vi "Elevator.vi"(8 "actuating axis":dbl, 11 "Elevator Locked?":bool) -> ()   [LabVIEW 2014]
uses:
  Robot Global Data.vi
panel:
  out "Winch Setpoint":dbl
  out "Winch Motor speed":dbl
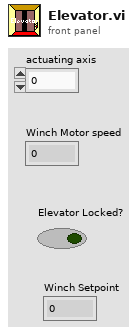
[diagram p1: front panel]
types:
  T1 = typedef "WPI_DigitalInputDevRef.ctl" = cluster{"DevStatus":errorcluster, "DIO Channel":T2, "Controller":T3}
  T2 = typedef "FPGA_DIOChannel.ctl" = enum8{"DIO 0", "DIO 1", "DIO 2", "DIO 3", "DIO 4", "DIO 5", "DIO 6", "DIO 7", "DIO 8", "DIO 9", "DIO MXP 0", "DIO MXP 1", "DIO MXP 2", "DIO MXP 3", "DIO MXP 4", "DIO MXP 5", "DIO MXP 6", "DIO MXP 7", "DIO MXP 8", "DIO MXP 9", "DIO MXP 10", "DIO MXP 11", "DIO MXP 12", "DIO MXP 13", "DIO MXP 14", "DIO MXP 15", "Invalid"}
  T3 = typedef "FPGA_TypedefDigitalModule.ctl" = enum16{"Controller 1"}
  T4 = typedef "WPI_MotorControlDeviceRef.ctl" = cluster{"DeviceStatus":errorcluster, "Type":T5, "PWM":cluster{"Controller":T3, "PWM Channel":T6, "DeadBand":T7}, "CAN":cluster{"Device Number":u8, "Control Mode":T8, "Semaphore":T9, "Max Vout":dbl, "TalonSRX Control Mode":T10}, "Invert":bool, "TransformRef":T11, "InvTransformRef":T11}
  T5 = typedef "WPI_MotorControlType.ctl" = enum16{"PWM", "CAN", "CANTalonSRX"}
  T6 = typedef "FPGA_DIOPWMChannel.ctl" = enum8{"PWM 0", "PWM 1", "PWM 2", "PWM 3", "PWM 4", "PWM 5", "PWM 6", "PWM 7", "PWM 8", "PWM 9", "PWM MXP 0", "PWM MXP 1", "PWM MXP 2", "PWM MXP 3", "PWM MXP 4", "PWM MXP 5", "PWM MXP 6", "PWM MXP 7", "PWM MXP 8", "PWM MXP 9", "Invalid"}
  T7 = typedef "WPI_PWMDeadband.ctl" = cluster{"Name":string, "maxPositivePwm":i32, "minPositivePwm":i32, "centerPwm":i32, "maxNegativePwm":i32, "minNegativePwm":i32, "angularRange":u16}
  T8 = typedef "WPI_CANJaguar_ControlMode.ctl" = enum8{"Percent VBus", "Current", "Speed", "Position", "Voltage"}
  T9 = typedef "Semaphore RefNum" = refnum<k1>
  T10 = typedef "WPI_CANTalonSRX_APIControlMode.ctl" = enum8{"Percent VBus", "Speed", "Position", "Slave", "Unchanged / Invalid"}
  T11 = typedef "WPI_PWMTransform_ConPane.ctl" = refnum<vi>
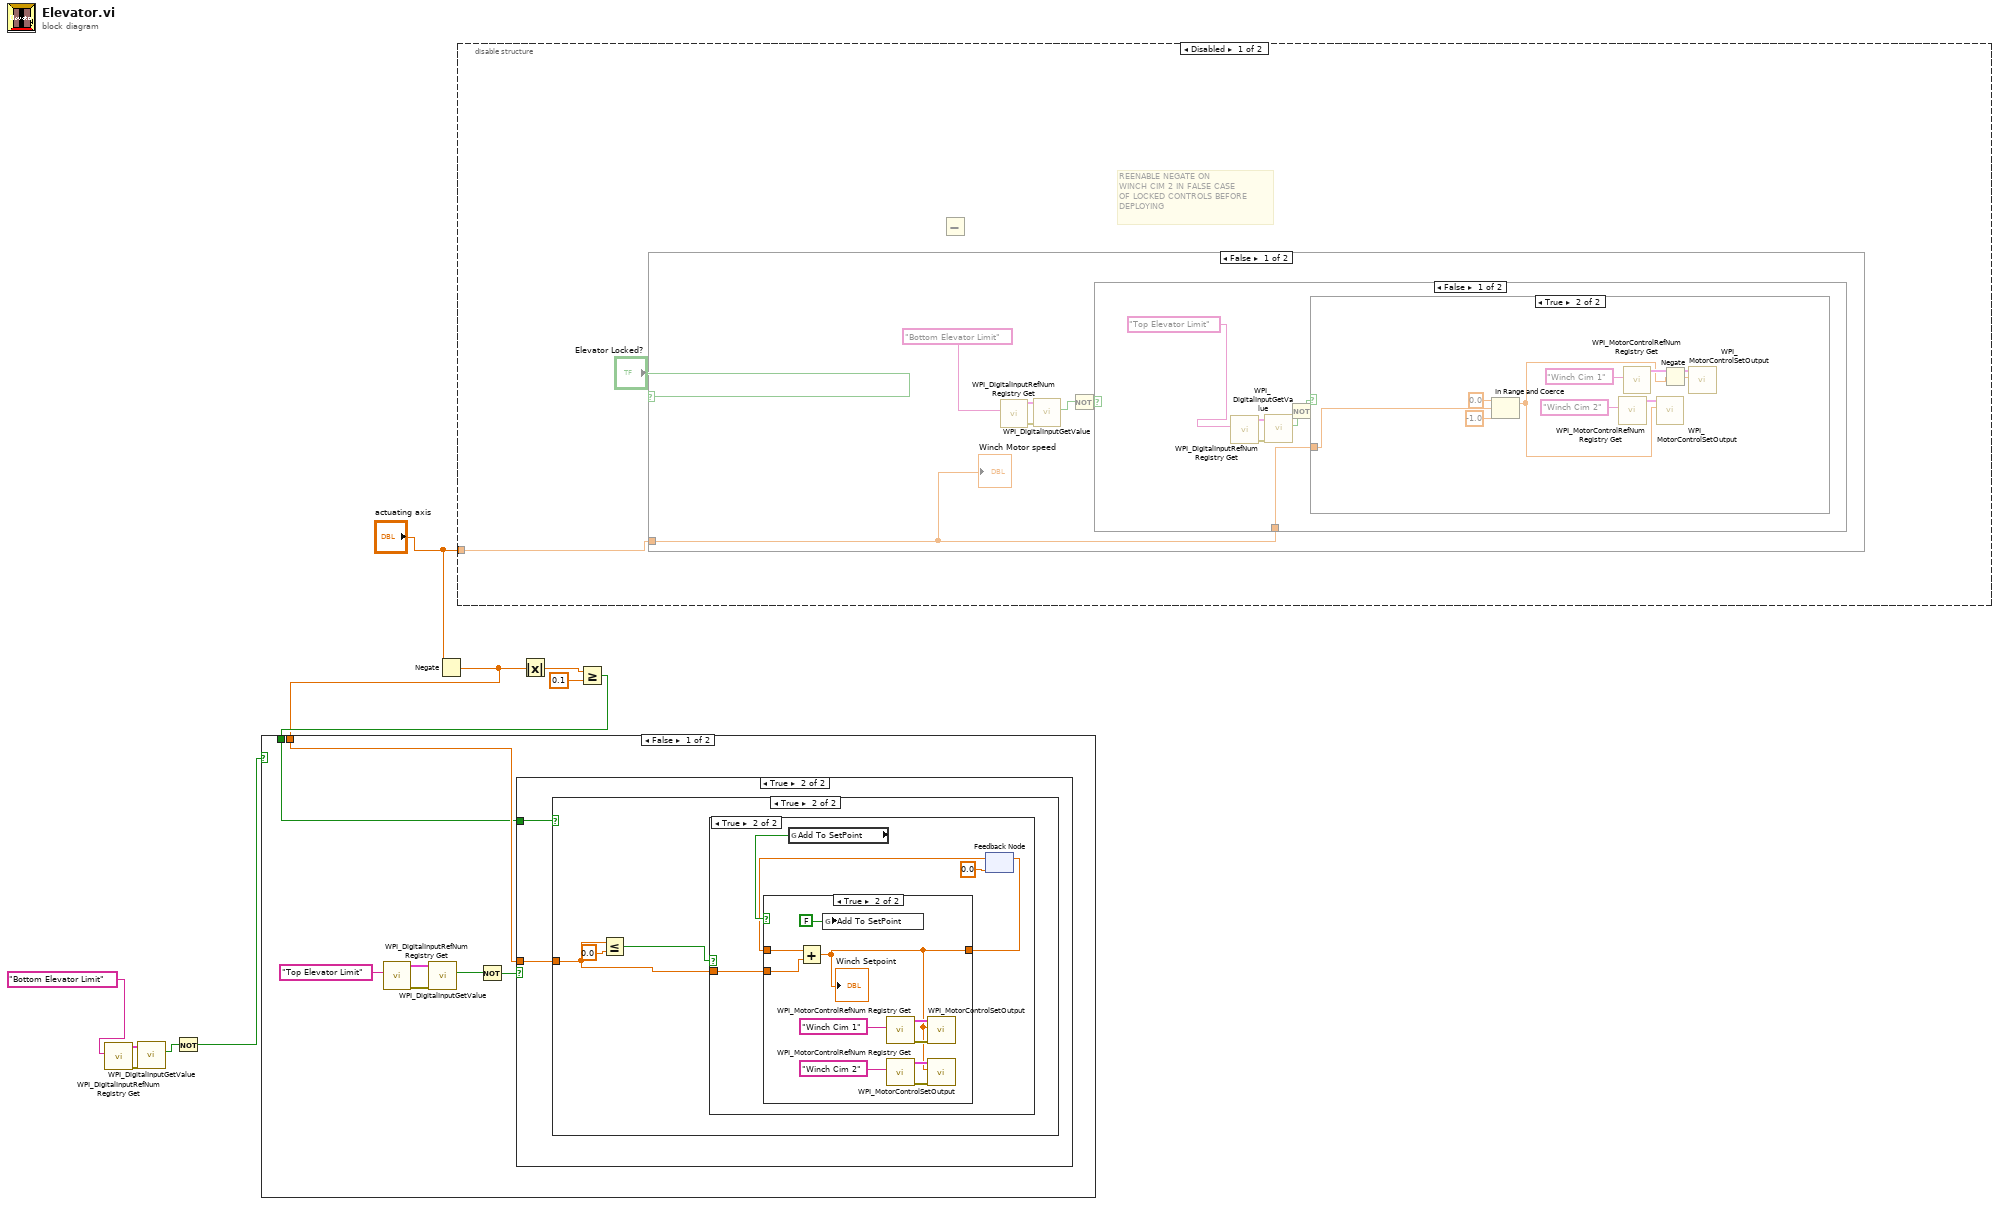
[diagram p0: block diagram]
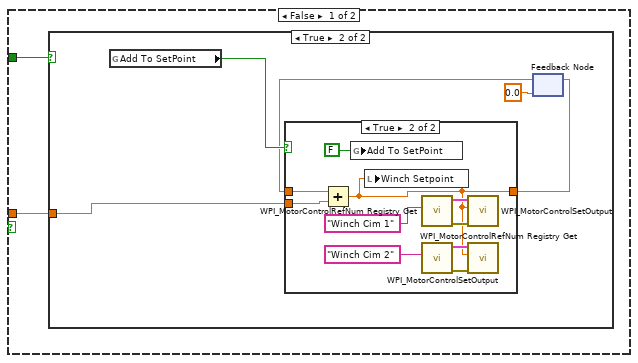
[diagram p2: hidden frame]
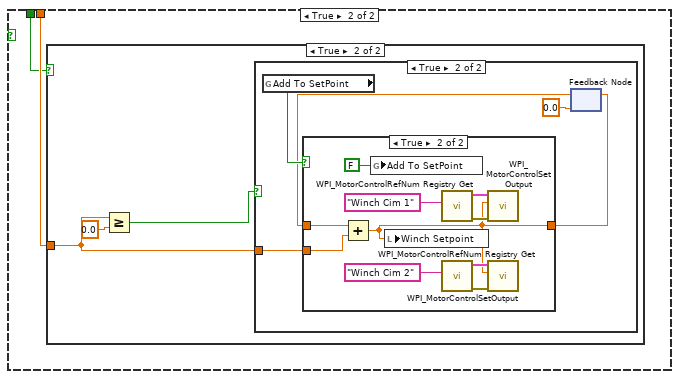
[diagram p8: hidden frame]
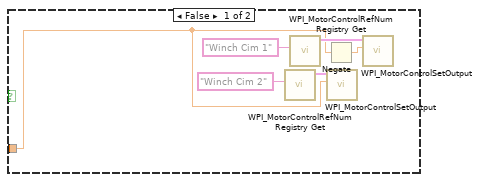
[diagram p12: hidden frame]
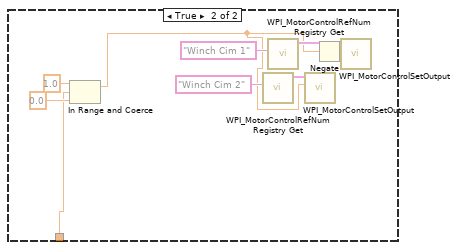
[diagram p13: hidden frame]
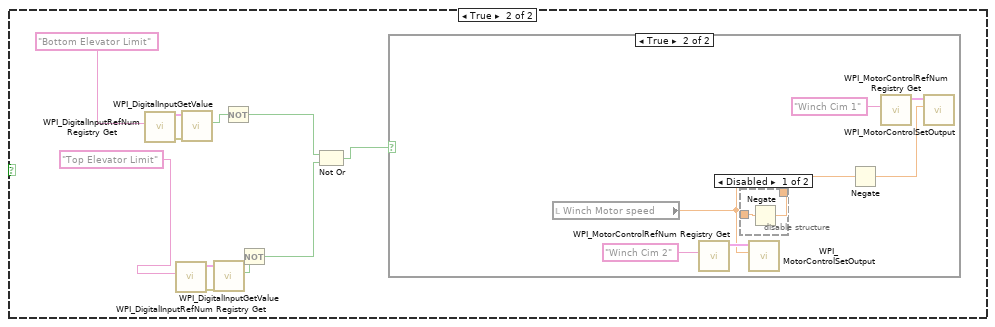
[diagram p14: hidden frame]
diagram:
  n1 = call <vilib>:"WPI_DigitalInputRefNum Registry Get.vi"("refnum name"="Bottom Elevator Limit") -> ("error out"=w8:errorcluster, "DigitalInputDevRef"=w7:T1)  [unwired: 9 in]
  n2 = call <vilib>:"WPI_DigitalInputGetValue.vi"("error in (no error)"=w8, "DigitalInputDevRef"=w7) -> ("Value"=w6:bool)  [unwired: 7 in, 2 out]
  n3 = Not(x=w6) -> (.not. x?=w5:bool)
  n4 = Negate(x="actuating axis") -> (-x=w1:dbl)
  n5 = disable-structure shown="Disabled" {
    disable-tunnel: "actuating axis" -> [w11 _]
    frame Disabled {
      # "REENABLE NEGATE ON\nWINCH CIM 2 IN FALSE CASE \nOF LOCKED CONTROLS BEFORE\nDEPLOYING"
      n6 = case shown="False" "Elevator Locked?" {
        tunnel: w11 -> [w13 _]
        frame False {
          n7 = call <vilib>:"WPI_DigitalInputRefNum Registry Get.vi"("refnum name"="Bottom Elevator Limit") -> ("error out"=w18:errorcluster, "DigitalInputDevRef"=w17:T1)  [unwired: 9 in]
          n8 = call <vilib>:"WPI_DigitalInputGetValue.vi"("error in (no error)"=w18, "DigitalInputDevRef"=w17) -> ("Value"=w16:bool)  [unwired: 7 in, 2 out]
          n9 = Not(x=w16) -> (.not. x?=w15:bool)
          n10 = case shown="False" w15 {
            tunnel: w13 -> [w20 w41]
            frame False {
              n11 = call <vilib>:"WPI_DigitalInputRefNum Registry Get.vi"("refnum name"="Top Elevator Limit") -> ("error out"=w23:errorcluster, "DigitalInputDevRef"=w24:T1)  [unwired: 9 in]
              n12 = call <vilib>:"WPI_DigitalInputGetValue.vi"("error in (no error)"=w23, "DigitalInputDevRef"=w24) -> ("Value"=w22:bool)  [unwired: 7 in, 2 out]
              n13 = Not(x=w22) -> (.not. x?=w21:bool)
              n14 = case shown="True" w21 {
                tunnel: w20 -> [w25 w32]
                frame False {
                  n15 = call <vilib>:"WPI_MotorControlRefNum Registry Get.vi"("refnum name"="Winch Cim 2" ("Name")) -> ("MotorControlDevRef"=w29:T4)  [unwired: 9 in, 1 out]
                  n16 = call <vilib>:"WPI_MotorControlRefNum Registry Get.vi"("refnum name"="Winch Cim 1" ("Name")) -> ("MotorControlDevRef"=w27:T4)  [unwired: 9 in, 1 out]
                  n17 = Negate(x=w25) -> (-x=w26:dbl)
                  n18 = call <vilib>:"WPI_MotorControlSetOutput.vi"("Output"=w25, "MotorControlDevRef"=w29) -> ()  [unwired: 7 in, 3 out]
                  n19 = call <vilib>:"WPI_MotorControlSetOutput.vi"("Output"=w26, "MotorControlDevRef"=w27) -> ()  [unwired: 7 in, 3 out]
                }
                frame True {
                  n20 = In Range and Coerce(upper limit=0.0, x=w32, lower limit=-1.0) -> (coerced(x)=w33:dbl)  [unwired: 1 out]
                  n21 = call <vilib>:"WPI_MotorControlRefNum Registry Get.vi"("refnum name"="Winch Cim 2" ("Name")) -> ("MotorControlDevRef"=w36:T4)  [unwired: 9 in, 1 out]
                  n22 = call <vilib>:"WPI_MotorControlRefNum Registry Get.vi"("refnum name"="Winch Cim 1" ("Name")) -> ("MotorControlDevRef"=w34:T4)  [unwired: 9 in, 1 out]
                  n23 = call <vilib>:"WPI_MotorControlSetOutput.vi"("Output"=w33, "MotorControlDevRef"=w36) -> ()  [unwired: 7 in, 3 out]
                  n24 = Negate(x=w33) -> (-x=w31:dbl)
                  n25 = call <vilib>:"WPI_MotorControlSetOutput.vi"("Output"=w31, "MotorControlDevRef"=w34) -> ()  [unwired: 7 in, 3 out]
                }
              }
            }
            frame True {
              n26 = In Range and Coerce(upper limit=1.0, x=w41, lower limit=0.0) -> (coerced(x)=w42:dbl)  [unwired: 1 out]
              n27 = call <vilib>:"WPI_MotorControlRefNum Registry Get.vi"("refnum name"="Winch Cim 2" ("Name")) -> ("MotorControlDevRef"=w45:T4)  [unwired: 9 in, 1 out]
              n28 = call <vilib>:"WPI_MotorControlRefNum Registry Get.vi"("refnum name"="Winch Cim 1" ("Name")) -> ("MotorControlDevRef"=w43:T4)  [unwired: 9 in, 1 out]
              n29 = call <vilib>:"WPI_MotorControlSetOutput.vi"("Output"=w42, "MotorControlDevRef"=w45) -> ()  [unwired: 7 in, 3 out]
              n30 = Negate(x=w42) -> (-x=w40:dbl)
              n31 = call <vilib>:"WPI_MotorControlSetOutput.vi"("Output"=w40, "MotorControlDevRef"=w43) -> ()  [unwired: 7 in, 3 out]
            }
          }
          "Winch Motor speed" <- w13
        }
        frame True {
          n32 = call <vilib>:"WPI_DigitalInputRefNum Registry Get.vi"("refnum name"="Bottom Elevator Limit") -> ("error out"=w59:errorcluster, "DigitalInputDevRef"=w58:T1)  [unwired: 9 in]
          n33 = call <vilib>:"WPI_DigitalInputRefNum Registry Get.vi"("refnum name"="Top Elevator Limit") -> ("error out"=w54:errorcluster, "DigitalInputDevRef"=w55:T1)  [unwired: 9 in]
          n34 = call <vilib>:"WPI_DigitalInputGetValue.vi"("error in (no error)"=w59, "DigitalInputDevRef"=w58) -> ("Value"=w57:bool)  [unwired: 7 in, 2 out]
          n35 = call <vilib>:"WPI_DigitalInputGetValue.vi"("error in (no error)"=w54, "DigitalInputDevRef"=w55) -> ("Value"=w53:bool)  [unwired: 7 in, 2 out]
          n36 = Not(x=w57) -> (.not. x?=w51:bool)
          n37 = Not(x=w53) -> (.not. x?=w50:bool)
          n38 = Not Or(1:w50, 2:w51) -> (0:w49:bool)
          n39 = case shown="True" w49 {
            frame False {
            }
            frame True {
              n40 = local read "Winch Motor speed"() -> (w61:dbl)
              n41 = call <vilib>:"WPI_MotorControlRefNum Registry Get.vi"("refnum name"="Winch Cim 2" ("Name")) -> ("MotorControlDevRef"=w64:T4)  [unwired: 9 in, 1 out]
              n42 = disable-structure shown="Disabled" {
                disable-tunnel: [w67 _] -> _
                disable-tunnel: _ -> [w66 _]
                frame Disabled {
                  n43 = Negate(x=w66) -> (-x=w67:dbl)
                }
                frame Enabled {
                }
              }
              n44 = call <vilib>:"WPI_MotorControlSetOutput.vi"("Output"=w61, "MotorControlDevRef"=w64) -> ()  [unwired: 7 in, 3 out]
              n45 = Negate(x=w61) -> (-x=w60:dbl)
              n46 = call <vilib>:"WPI_MotorControlRefNum Registry Get.vi"("refnum name"="Winch Cim 1" ("Name")) -> ("MotorControlDevRef"=w62:T4)  [unwired: 9 in, 1 out]
              n47 = call <vilib>:"WPI_MotorControlSetOutput.vi"("Output"=w60, "MotorControlDevRef"=w62) -> ()  [unwired: 7 in, 3 out]
            }
          }
        }
      }
      n48 = Subtract() -> ()  [unwired: 2 in, 1 out]
    }
    frame Enabled {
    }
  }
  n49 = Absolute Value(x=w1) -> (abs(x)=w9:dbl)
  n50 = Greater Or Equal?(x=w9, y=0.1) -> (x >= y?=w3:bool)
  n51 = case shown="False" w5 {
    tunnel: w1 -> [w70 w115]
    tunnel: w3 -> [w69 w114]
    frame False {
      n52 = call <vilib>:"WPI_DigitalInputRefNum Registry Get.vi"("refnum name"="Top Elevator Limit") -> ("error out"=w73:errorcluster, "DigitalInputDevRef"=w74:T1)  [unwired: 9 in]
      n53 = call <vilib>:"WPI_DigitalInputGetValue.vi"("error in (no error)"=w73, "DigitalInputDevRef"=w74) -> ("Value"=w71:bool)  [unwired: 7 in, 2 out]
      n54 = Not(x=w71) -> (.not. x?=w68:bool)
      n55 = case shown="True" w68 {
        tunnel: w70 -> [w76 w94]
        tunnel: w69 -> [w75 w93]
        frame False {
          n56 = case shown="True" w75 {
            tunnel: w76 -> [_ w77]
            frame False {
            }
            frame True {
              n57 = global read "Robot Global Data.vi" "Add To SetPoint"() -> (w81:bool)
              n58 = feedback #1(0.0) -> (w79:dbl)
              n59 = case shown="True" w81 {
                tunnel: w79 -> [w82 w91]
                tunnel: w77 -> [_ w92]
                tunnel: [w82 w83] -> w78
                frame False {
                }
                frame True {
                  n60 = Add(x=w91, y=w92) -> (x+y=w83:dbl)
                  n61 = global write "Robot Global Data.vi" "Add To SetPoint"(FALSE) -> ()
                  n62 = local write "Winch Setpoint"(w83) -> ()
                  n63 = call <vilib>:"WPI_MotorControlRefNum Registry Get.vi"("refnum name"="Winch Cim 1" ("Name")) -> ("error out"=w88:errorcluster, "MotorControlDevRef"=w89:T4)  [unwired: 9 in]
                  n64 = call <vilib>:"WPI_MotorControlRefNum Registry Get.vi"("refnum name"="Winch Cim 2" ("Name")) -> ("error out"=w85:errorcluster, "MotorControlDevRef"=w86:T4)  [unwired: 9 in]
                  n65 = call <vilib>:"WPI_MotorControlSetOutput.vi"("error in (no error)"=w88, "Output"=w83, "MotorControlDevRef"=w89) -> ()  [unwired: 6 in, 3 out]
                  n66 = call <vilib>:"WPI_MotorControlSetOutput.vi"("error in (no error)"=w85, "Output"=w83, "MotorControlDevRef"=w86) -> ()  [unwired: 6 in, 3 out]
                }
              }
              n67 = feedback-in #1(w78) -> ()
            }
          }
        }
        frame True {
          n68 = case shown="True" w93 {
            tunnel: w94 -> [_ w96]
            frame False {
            }
            frame True {
              n69 = Less Or Equal?(x=w96, y=0.0) -> (x <= y?=w95:bool)
              n70 = case shown="True" w95 {
                tunnel: w96 -> [_ w98]
                frame False {
                }
                frame True {
                  n71 = global read "Robot Global Data.vi" "Add To SetPoint"() -> (w102:bool)
                  n72 = feedback #2(0.0) -> (w100:dbl)
                  n73 = case shown="True" w102 {
                    tunnel: w100 -> [w103 w113]
                    tunnel: [w103 w105] -> w99
                    tunnel: w98 -> [_ w104]
                    frame False {
                    }
                    frame True {
                      n74 = Add(x=w113, y=w104) -> (x+y=w105:dbl)
                      "Winch Setpoint" <- w105
                      n75 = global write "Robot Global Data.vi" "Add To SetPoint"(FALSE) -> ()
                      n76 = call <vilib>:"WPI_MotorControlRefNum Registry Get.vi"("refnum name"="Winch Cim 1" ("Name")) -> ("error out"=w110:errorcluster, "MotorControlDevRef"=w111:T4)  [unwired: 9 in]
                      n77 = call <vilib>:"WPI_MotorControlRefNum Registry Get.vi"("refnum name"="Winch Cim 2" ("Name")) -> ("error out"=w107:errorcluster, "MotorControlDevRef"=w108:T4)  [unwired: 9 in]
                      n78 = call <vilib>:"WPI_MotorControlSetOutput.vi"("error in (no error)"=w110, "Output"=w105, "MotorControlDevRef"=w111) -> ()  [unwired: 6 in, 3 out]
                      n79 = call <vilib>:"WPI_MotorControlSetOutput.vi"("error in (no error)"=w107, "Output"=w105, "MotorControlDevRef"=w108) -> ()  [unwired: 6 in, 3 out]
                    }
                  }
                  n80 = feedback-in #2(w99) -> ()
                }
              }
            }
          }
        }
      }
    }
    frame True {
      n81 = case shown="True" w114 {
        tunnel: w115 -> [_ w116]
        frame False {
        }
        frame True {
          n82 = Greater Or Equal?(x=w116, y=0.0) -> (x >= y?=w117:bool)
          n83 = case shown="True" w117 {
            tunnel: w116 -> [_ w119]
            frame False {
            }
            frame True {
              n84 = global read "Robot Global Data.vi" "Add To SetPoint"() -> (w123:bool)
              n85 = feedback #3(0.0) -> (w121:dbl)
              n86 = case shown="True" w123 {
                tunnel: w121 -> [w124 w134]
                tunnel: [w124 w126] -> w120
                tunnel: w119 -> [_ w125]
                frame False {
                }
                frame True {
                  n87 = Add(x=w134, y=w125) -> (x+y=w126:dbl)
                  n88 = global write "Robot Global Data.vi" "Add To SetPoint"(FALSE) -> ()
                  n89 = local write "Winch Setpoint"(w126) -> ()
                  n90 = call <vilib>:"WPI_MotorControlRefNum Registry Get.vi"("refnum name"="Winch Cim 1" ("Name")) -> ("error out"=w131:errorcluster, "MotorControlDevRef"=w132:T4)  [unwired: 9 in]
                  n91 = call <vilib>:"WPI_MotorControlRefNum Registry Get.vi"("refnum name"="Winch Cim 2" ("Name")) -> ("error out"=w128:errorcluster, "MotorControlDevRef"=w129:T4)  [unwired: 9 in]
                  n92 = call <vilib>:"WPI_MotorControlSetOutput.vi"("error in (no error)"=w131, "Output"=w126, "MotorControlDevRef"=w132) -> ()  [unwired: 6 in, 3 out]
                  n93 = call <vilib>:"WPI_MotorControlSetOutput.vi"("error in (no error)"=w128, "Output"=w126, "MotorControlDevRef"=w129) -> ()  [unwired: 6 in, 3 out]
                }
              }
              n94 = feedback-in #3(w120) -> ()
            }
          }
        }
      }
    }
  }
